vi "Count Command Errors1.vi"(8 "error in (no error)":errorcluster) -> (0 "error out":errorcluster, 3 "Command Errors":i32)   [LabVIEW 2020]
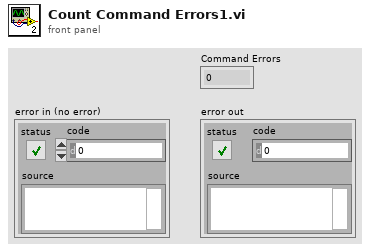
[diagram p1: front panel]
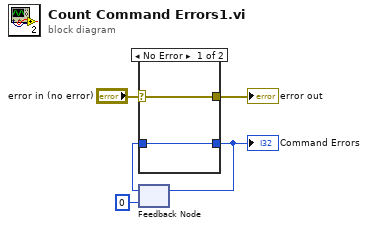
[diagram p0: block diagram]
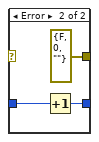
[diagram p2: hidden frame]
diagram:
  n1 = feedback #1(0) -> (w3:i32)
  n2 = case shown="No Error" "error in (no error)" {
    selector: "error in (no error)" -> [w6 _]
    tunnel: w3 -> [w7 w10]
    tunnel: [w7 w9] -> w2
    tunnel: [w6 errorcluster {"status"=FALSE, "code"=0, "source"=""} ("error IO")] -> w5
    frame No Error {
    }
    frame Error {
      n3 = Increment(x=w10) -> (x+1=w9:i32)
    }
  }
  "Command Errors" <- w2
  "error out" <- w5
  n4 = feedback-in #1(w2) -> ()
